vi "Distributor - SET - Triggered Event.vi"(8 "error in (no error)":errorcluster, 10 "Events":T1, 11 "Parent_Class in":refnum<class "Message_Distributor_Class.lvclass">) -> (0 "error out":errorcluster, 3 "Parent_Class out":refnum<class "Message_Distributor_Class.lvclass">)   [LabVIEW 2023, in "Actor_Message_Distributor.lvlib" / "Message_Distributor_Class.lvclass"]
uses:
  Message_Distributor_Class.lvclass
  Usr Ev/Distributor - Ctrl - Enum - Events.ctl
  Message_Distributor_Class.lvclass/Message_Distributor_Class.ctl
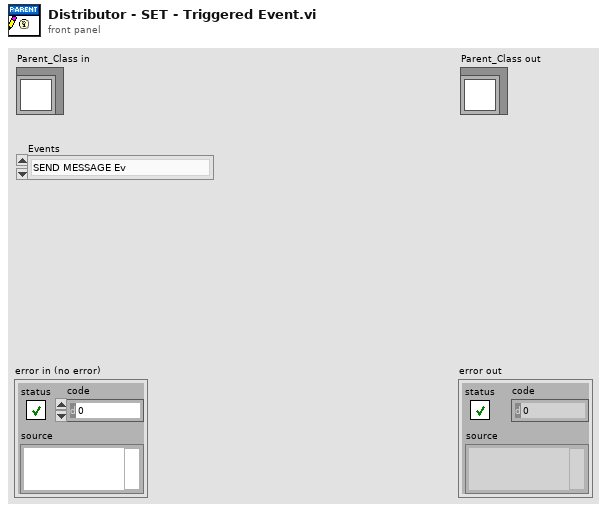
[diagram p1: front panel]
types:
  T1 = typedef "Actor_Message_Distributor.lvlib/Message_Distributor_Class.lvclass/Distributor - Ctrl - Enum - Events.ctl" = enum16{"SEND MESSAGE Ev", "STOP_ACTOR Ev", "INIT_ACTOR Ev", "START Ev", "STOP Ev", "GET Ev", "SET Ev", "ERROR_HANDLER Ev", "RESET Ev", "DISPATCH MESSAGE 2 CHILDS Ev", "ECU RESET Ev"}
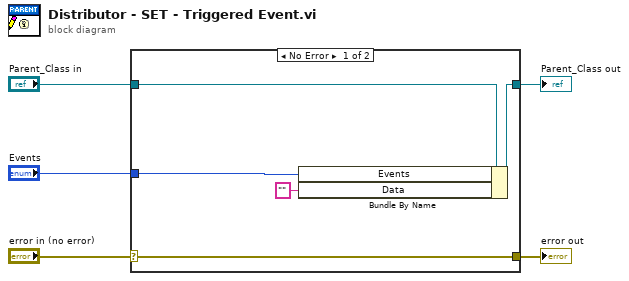
[diagram p0: block diagram]
diagram:
  n1 = case shown="No Error" "error in (no error)" {
    selector: "error in (no error)" -> [w10 w11]
    tunnel: [w10 w11] -> w4
    tunnel: [w8 w12] -> w2
    tunnel: "Parent_Class in" -> [w9 w12]
    tunnel: "Events" -> [w7 _]
    frame No Error {
      n2 = Bundle By Name(cluster=w9, "Events"=w7, "Data"="" ("Parent Trigger Event Cluster.Data")) -> (w8:refnum<class "Message_Distributor_Class.lvclass">)
    }
    frame Error {
    }
  }
  "error out" <- w4
  "Parent_Class out" <- w2
